vi "EventLogger.FlushToDisk.vi"(8 "error in":errorcluster) -> (0 "error out":errorcluster)   [LabVIEW 2019, in "Tools.lvlib"]
uses:
  Tools.lvlib
  <vilib>/NI/Event Logger Library/EventLog/EventLog.lvclass
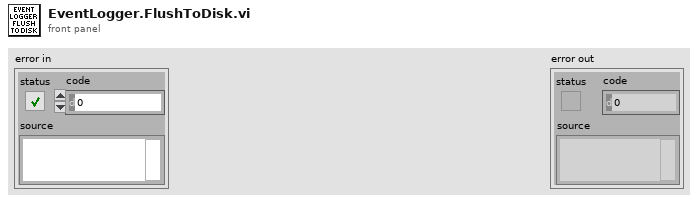
[diagram p1: front panel]
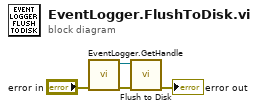
[diagram p0: block diagram]
diagram:
  n1 = call "EventLogger.GetHandle.vi"("error in"="error in") -> ("error out"=w2:errorcluster, "EventLog ref"=w1:refnum<class "EventLog.lvclass">)  [unwired: 9 in]
  n2 = call <vilib>:"Flush to Disk.vi"("error in (no error)"=w2, "EventLog ref"=w1) -> ("error out"=→"error out":errorcluster)  [unwired: 8 in, 1 out]
